vi "GenerateUniqueFilename.vi"(11 "Base Name":string) -> (3 "String":string)   [LabVIEW 2018]
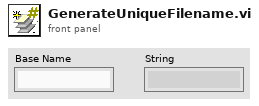
[diagram p1: front panel]
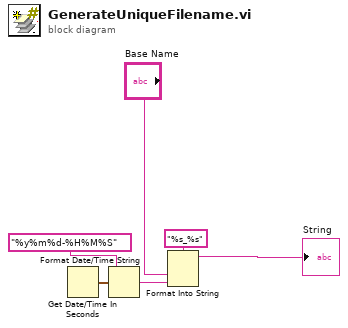
[diagram p0: block diagram]
diagram:
  n1 = Get Date/Time In Seconds() -> (seconds since 1Jan1904=w2:timestamp)
  n2 = Format Date/Time String(time format string (%c)="%y%m%d-%H%M%S", seconds (now)=w2) -> (date/time string=w3:string)  [unwired: 1 in]
  n3 = Format Into String(format string="%s_%s", "Base Name", w3) -> (resulting string=→"String":string)  [unwired: 2 in, 1 out]
